vi "四通道零漂采集1A4DEB1.vi"() -> ()   [LabVIEW 2011]
doc: "Use this template to build a producer/consumer design pattern. Use this template when you need to execute a process, such as data analysis, when a data source, such as a triggered acquisition, produces data at an uneven rate and you need to execute the process when the data becomes available."
uses:
  <vilib>/Utility/inputDevices.llb/closeKeyboard.vi
  <vilib>/Utility/inputDevices.llb/keyboardAcquire.vi
  <vilib>/Utility/file.llb/Write To Spreadsheet File (string).vi
  <vilib>/Utility/file.llb/Read From Spreadsheet File (string).vi
  <vilib>/Analysis/NI_AALBase.lvlib
panel:
  in  "每几秒采一个点":i32=1
  in  "计算零偏\n稳定性":bool
  out "零偏值4":dbl[unit]
  out "零偏稳定性4":dbl[unit]
  in  "灵敏度4":dbl[unit]
  out "standard deviation 4":dbl[unit] caption="标准差4" format="%.6f"
  out "mean 4":dbl[unit] caption="平均值4" format="%.6f"
  out "零偏值3":dbl[unit]
  out "零偏稳定性3":dbl[unit]
  in  "灵敏度3":dbl[unit]
  out "standard deviation 3":dbl[unit] caption="标准差3" format="%.6f"
  out "mean 3":dbl[unit] caption="平均值3" format="%.6f"
  out "零偏值2":dbl[unit]
  out "零偏稳定性2":dbl[unit]
  in  "灵敏度2":dbl[unit]
  out "standard deviation 2":dbl[unit] caption="标准差2" format="%.6f"
  out "mean 2":dbl[unit] caption="平均值2" format="%.6f"
  out "零偏值1":dbl[unit]
  out "零偏稳定性1":dbl[unit]
  in  "灵敏度1":dbl[unit]
  out "standard deviation":dbl[unit] caption="标准差1" format="%.6f"
  out "mean":dbl[unit] caption="平均值1" format="%.6f"
  out "0g输出值(V) 3":dbl
  out "0g输出值(V) 2":dbl
  out "0g输出值(V) 1":dbl
  out "a1通道零漂采集":dbl(graph)
  out "a3通道零漂采集":dbl(graph)
  out "a2通道零漂采集":dbl(graph)
  in  "删除文件":bool
  in  "打开文件":bool
  in  "创建文件":bool
  in  "开始采零漂":bool
  in  "打开采集卡":bool
  in  "闹钟定时":bool
  in  "时间标识":timestamp format="%<%H:%M\n%x>T"
  out "采集数据":string[][](array[string])
  out "点数":i16
  out "x":i16
  in  "传感器编号":string
  out "a0通道零漂采集":dbl(graph)
  out "0g输出值(V)":dbl
  in  "stop":bool
  # "四通道零漂采集测试"
  # "D"
  # "O"
  # "N"
  # "S"
  # "B"
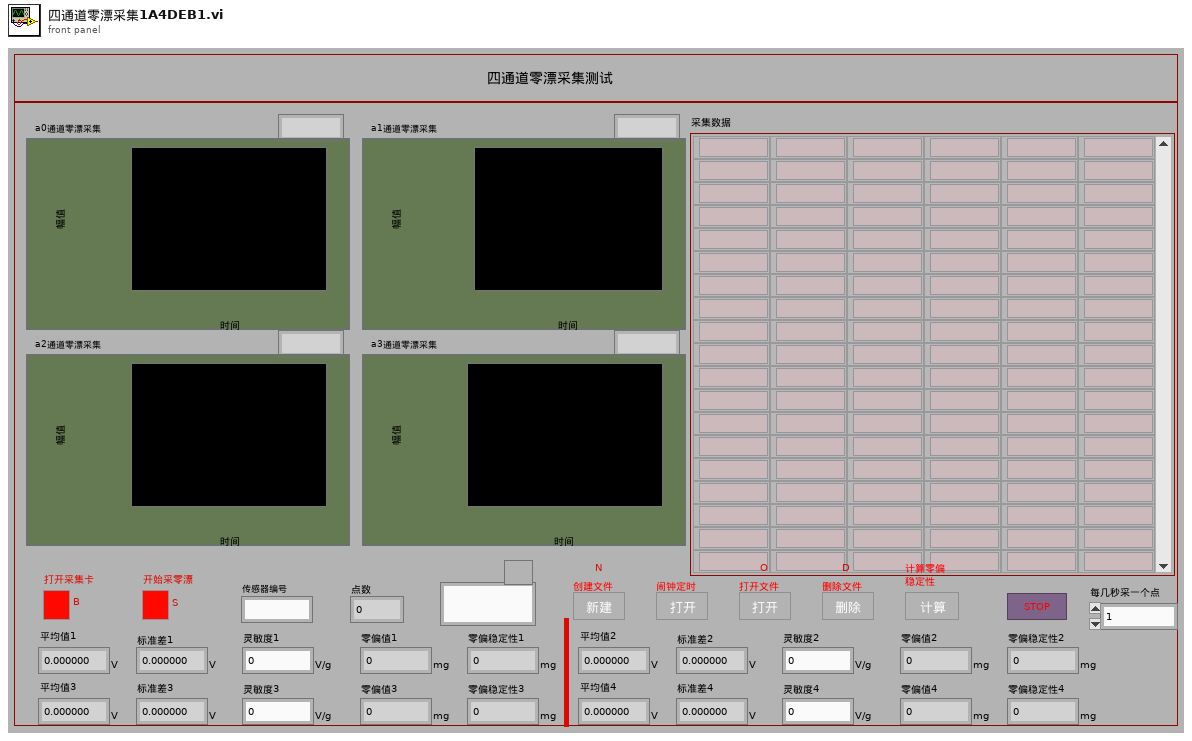
[diagram p1: front panel]
types:
  T1 = enum16{"0", "1", "2", "3", "4", "5", "6", "7", "8", "9", "A", "B", "C", "D", "E", "F", "G", "H", "I", "J", "K", "L", "M", "N", "O", "P", "Q", "R", "S", "T", "U", "V", "W", "X", "Y", "Z", "F1", "F2", "F3", "F4", "F5", "F6", "F7", "F8", "F9", "F10", "F11", "F12", "F13", "F14", "F15", "ADD", "BACK", "BACKSLASH", "CAPITAL", "COMMA", "DECIMAL", "DELETE", "DIVIDE", "DOWN", "END", "EQUALS", "ESCAPE", "GRAVE (`)", "HOME", "INSERT", "LBRACKET", "LCONTROL", "LEFT", "L ALT", "LSHIFT", "LWIN", "MINUS", "MULTIPLY", "NEXT", "NUMLOCK", "NUMPAD_0", "NUMPAD_1", "NUMPAD_2", "NUMPAD_3", "NUMPAD_4", "NUMPAD_5", "NUMPAD_6", "NUMPAD_7", "NUMPAD_8", "NUMPAD_9", "PAUSE", "PERIOD", "PRIOR (PG UP)", "RBRACKET", "RCONTROL", "RETURN", "RIGHT", "R ALT", "RSHIFT", "RWIN", "SCROLL", "SEMICOLON", "SLASH", "SPACE", "SUBTRACT", "TAB", "UP", "ENTER (num pad)", "' (quote)"}
  T2 = enum16{"0", "1", "2", "3", "4", "5", "6", "7", "8", "9", "A", "B", "C", "D", "E", "F", "G", "H", "I", "J", "K", "L", "M", "N", "O", "P", "Q", "R", "S", "T", "U", "V", "W", "X", "Y", "Z", "F1", "F2", "F3", "F4", "F5", "F6", "F7", "F8", "F9", "F10", "F11", "F12", "F13", "F14", "F15", "ADD", "BACK", "BACKSLASH", "CAPITAL", "COMMA", "DECIMAL", "DELETE", "DIVIDE", "DOWN", "END", "EQUALS", "ESCAPE", "GRAVE (`)", "HOME", "INSERT", "LBRACKET", "LCONTROL", "LEFT", "L ALT", "LSHIFT", "LWIN", "MINUS", "MULTIPLY", "NEXT", "NUMLOCK", "NUMPAD_0", "NUMPAD_1", "NUMPAD_2", "NUMPAD_3", "NUMPAD_4", "NUMPAD_5", "NUMPAD_6", "NUMPAD_7", "NUMPAD_8", "NUMPAD_9", "PAUSE", "PERIOD", "PRIOR (PG UP)", "RBRACKET", "RCONTROL", "RETURN", "RIGHT", "R ALT", "RSHIFT", "RWIN", "SCROLL", "SEMICOLON", "SLASH", "SPACE", "SUBTRACT", "TAB", "UP", "ENTER (num pad)", "' (quote)"}[]
  T3 = cluster{"keys pressed[0]":enum16{"0", "1", "2", "3", "4", "5", "6", "7", "8", "9", "A", "B", "C", "D", "E", "F", "G", "H", "I", "J", "K", "L", "M", "N", "O", "P", "Q", "R", "S", "T", "U", "V", "W", "X", "Y", "Z", "F1", "F2", "F3", "F4", "F5", "F6", "F7", "F8", "F9", "F10", "F11", "F12", "F13", "F14", "F15", "ADD", "BACK", "BACKSLASH", "CAPITAL", "COMMA", "DECIMAL", "DELETE", "DIVIDE", "DOWN", "END", "EQUALS", "ESCAPE", "GRAVE (`)", "HOME", "INSERT", "LBRACKET", "LCONTROL", "LEFT", "L ALT", "LSHIFT", "LWIN", "MINUS", "MULTIPLY", "NEXT", "NUMLOCK", "NUMPAD_0", "NUMPAD_1", "NUMPAD_2", "NUMPAD_3", "NUMPAD_4", "NUMPAD_5", "NUMPAD_6", "NUMPAD_7", "NUMPAD_8", "NUMPAD_9", "PAUSE", "PERIOD", "PRIOR (PG UP)", "RBRACKET", "RCONTROL", "RETURN", "RIGHT", "R ALT", "RSHIFT", "RWIN", "SCROLL", "SEMICOLON", "SLASH", "SPACE", "SUBTRACT", "TAB", "UP", "ENTER (num pad)", "' (quote)"}, "keys pressed[1]":enum16{"0", "1", "2", "3", "4", "5", "6", "7", "8", "9", "A", "B", "C", "D", "E", "F", "G", "H", "I", "J", "K", "L", "M", "N", "O", "P", "Q", "R", "S", "T", "U", "V", "W", "X", "Y", "Z", "F1", "F2", "F3", "F4", "F5", "F6", "F7", "F8", "F9", "F10", "F11", "F12", "F13", "F14", "F15", "ADD", "BACK", "BACKSLASH", "CAPITAL", "COMMA", "DECIMAL", "DELETE", "DIVIDE", "DOWN", "END", "EQUALS", "ESCAPE", "GRAVE (`)", "HOME", "INSERT", "LBRACKET", "LCONTROL", "LEFT", "L ALT", "LSHIFT", "LWIN", "MINUS", "MULTIPLY", "NEXT", "NUMLOCK", "NUMPAD_0", "NUMPAD_1", "NUMPAD_2", "NUMPAD_3", "NUMPAD_4", "NUMPAD_5", "NUMPAD_6", "NUMPAD_7", "NUMPAD_8", "NUMPAD_9", "PAUSE", "PERIOD", "PRIOR (PG UP)", "RBRACKET", "RCONTROL", "RETURN", "RIGHT", "R ALT", "RSHIFT", "RWIN", "SCROLL", "SEMICOLON", "SLASH", "SPACE", "SUBTRACT", "TAB", "UP", "ENTER (num pad)", "' (quote)"}, "keys pressed[2]":enum16{"0", "1", "2", "3", "4", "5", "6", "7", "8", "9", "A", "B", "C", "D", "E", "F", "G", "H", "I", "J", "K", "L", "M", "N", "O", "P", "Q", "R", "S", "T", "U", "V", "W", "X", "Y", "Z", "F1", "F2", "F3", "F4", "F5", "F6", "F7", "F8", "F9", "F10", "F11", "F12", "F13", "F14", "F15", "ADD", "BACK", "BACKSLASH", "CAPITAL", "COMMA", "DECIMAL", "DELETE", "DIVIDE", "DOWN", "END", "EQUALS", "ESCAPE", "GRAVE (`)", "HOME", "INSERT", "LBRACKET", "LCONTROL", "LEFT", "L ALT", "LSHIFT", "LWIN", "MINUS", "MULTIPLY", "NEXT", "NUMLOCK", "NUMPAD_0", "NUMPAD_1", "NUMPAD_2", "NUMPAD_3", "NUMPAD_4", "NUMPAD_5", "NUMPAD_6", "NUMPAD_7", "NUMPAD_8", "NUMPAD_9", "PAUSE", "PERIOD", "PRIOR (PG UP)", "RBRACKET", "RCONTROL", "RETURN", "RIGHT", "R ALT", "RSHIFT", "RWIN", "SCROLL", "SEMICOLON", "SLASH", "SPACE", "SUBTRACT", "TAB", "UP", "ENTER (num pad)", "' (quote)"}, "keys pressed[3]":enum16{"0", "1", "2", "3", "4", "5", "6", "7", "8", "9", "A", "B", "C", "D", "E", "F", "G", "H", "I", "J", "K", "L", "M", "N", "O", "P", "Q", "R", "S", "T", "U", "V", "W", "X", "Y", "Z", "F1", "F2", "F3", "F4", "F5", "F6", "F7", "F8", "F9", "F10", "F11", "F12", "F13", "F14", "F15", "ADD", "BACK", "BACKSLASH", "CAPITAL", "COMMA", "DECIMAL", "DELETE", "DIVIDE", "DOWN", "END", "EQUALS", "ESCAPE", "GRAVE (`)", "HOME", "INSERT", "LBRACKET", "LCONTROL", "LEFT", "L ALT", "LSHIFT", "LWIN", "MINUS", "MULTIPLY", "NEXT", "NUMLOCK", "NUMPAD_0", "NUMPAD_1", "NUMPAD_2", "NUMPAD_3", "NUMPAD_4", "NUMPAD_5", "NUMPAD_6", "NUMPAD_7", "NUMPAD_8", "NUMPAD_9", "PAUSE", "PERIOD", "PRIOR (PG UP)", "RBRACKET", "RCONTROL", "RETURN", "RIGHT", "R ALT", "RSHIFT", "RWIN", "SCROLL", "SEMICOLON", "SLASH", "SPACE", "SUBTRACT", "TAB", "UP", "ENTER (num pad)", "' (quote)"}, "keys pressed[4]":enum16{"0", "1", "2", "3", "4", "5", "6", "7", "8", "9", "A", "B", "C", "D", "E", "F", "G", "H", "I", "J", "K", "L", "M", "N", "O", "P", "Q", "R", "S", "T", "U", "V", "W", "X", "Y", "Z", "F1", "F2", "F3", "F4", "F5", "F6", "F7", "F8", "F9", "F10", "F11", "F12", "F13", "F14", "F15", "ADD", "BACK", "BACKSLASH", "CAPITAL", "COMMA", "DECIMAL", "DELETE", "DIVIDE", "DOWN", "END", "EQUALS", "ESCAPE", "GRAVE (`)", "HOME", "INSERT", "LBRACKET", "LCONTROL", "LEFT", "L ALT", "LSHIFT", "LWIN", "MINUS", "MULTIPLY", "NEXT", "NUMLOCK", "NUMPAD_0", "NUMPAD_1", "NUMPAD_2", "NUMPAD_3", "NUMPAD_4", "NUMPAD_5", "NUMPAD_6", "NUMPAD_7", "NUMPAD_8", "NUMPAD_9", "PAUSE", "PERIOD", "PRIOR (PG UP)", "RBRACKET", "RCONTROL", "RETURN", "RIGHT", "R ALT", "RSHIFT", "RWIN", "SCROLL", "SEMICOLON", "SLASH", "SPACE", "SUBTRACT", "TAB", "UP", "ENTER (num pad)", "' (quote)"}, "keys pressed[5]":enum16{"0", "1", "2", "3", "4", "5", "6", "7", "8", "9", "A", "B", "C", "D", "E", "F", "G", "H", "I", "J", "K", "L", "M", "N", "O", "P", "Q", "R", "S", "T", "U", "V", "W", "X", "Y", "Z", "F1", "F2", "F3", "F4", "F5", "F6", "F7", "F8", "F9", "F10", "F11", "F12", "F13", "F14", "F15", "ADD", "BACK", "BACKSLASH", "CAPITAL", "COMMA", "DECIMAL", "DELETE", "DIVIDE", "DOWN", "END", "EQUALS", "ESCAPE", "GRAVE (`)", "HOME", "INSERT", "LBRACKET", "LCONTROL", "LEFT", "L ALT", "LSHIFT", "LWIN", "MINUS", "MULTIPLY", "NEXT", "NUMLOCK", "NUMPAD_0", "NUMPAD_1", "NUMPAD_2", "NUMPAD_3", "NUMPAD_4", "NUMPAD_5", "NUMPAD_6", "NUMPAD_7", "NUMPAD_8", "NUMPAD_9", "PAUSE", "PERIOD", "PRIOR (PG UP)", "RBRACKET", "RCONTROL", "RETURN", "RIGHT", "R ALT", "RSHIFT", "RWIN", "SCROLL", "SEMICOLON", "SLASH", "SPACE", "SUBTRACT", "TAB", "UP", "ENTER (num pad)", "' (quote)"}, "keys pressed[6]":enum16{"0", "1", "2", "3", "4", "5", "6", "7", "8", "9", "A", "B", "C", "D", "E", "F", "G", "H", "I", "J", "K", "L", "M", "N", "O", "P", "Q", "R", "S", "T", "U", "V", "W", "X", "Y", "Z", "F1", "F2", "F3", "F4", "F5", "F6", "F7", "F8", "F9", "F10", "F11", "F12", "F13", "F14", "F15", "ADD", "BACK", "BACKSLASH", "CAPITAL", "COMMA", "DECIMAL", "DELETE", "DIVIDE", "DOWN", "END", "EQUALS", "ESCAPE", "GRAVE (`)", "HOME", "INSERT", "LBRACKET", "LCONTROL", "LEFT", "L ALT", "LSHIFT", "LWIN", "MINUS", "MULTIPLY", "NEXT", "NUMLOCK", "NUMPAD_0", "NUMPAD_1", "NUMPAD_2", "NUMPAD_3", "NUMPAD_4", "NUMPAD_5", "NUMPAD_6", "NUMPAD_7", "NUMPAD_8", "NUMPAD_9", "PAUSE", "PERIOD", "PRIOR (PG UP)", "RBRACKET", "RCONTROL", "RETURN", "RIGHT", "R ALT", "RSHIFT", "RWIN", "SCROLL", "SEMICOLON", "SLASH", "SPACE", "SUBTRACT", "TAB", "UP", "ENTER (num pad)", "' (quote)"}, "keys pressed[7]":enum16{"0", "1", "2", "3", "4", "5", "6", "7", "8", "9", "A", "B", "C", "D", "E", "F", "G", "H", "I", "J", "K", "L", "M", "N", "O", "P", "Q", "R", "S", "T", "U", "V", "W", "X", "Y", "Z", "F1", "F2", "F3", "F4", "F5", "F6", "F7", "F8", "F9", "F10", "F11", "F12", "F13", "F14", "F15", "ADD", "BACK", "BACKSLASH", "CAPITAL", "COMMA", "DECIMAL", "DELETE", "DIVIDE", "DOWN", "END", "EQUALS", "ESCAPE", "GRAVE (`)", "HOME", "INSERT", "LBRACKET", "LCONTROL", "LEFT", "L ALT", "LSHIFT", "LWIN", "MINUS", "MULTIPLY", "NEXT", "NUMLOCK", "NUMPAD_0", "NUMPAD_1", "NUMPAD_2", "NUMPAD_3", "NUMPAD_4", "NUMPAD_5", "NUMPAD_6", "NUMPAD_7", "NUMPAD_8", "NUMPAD_9", "PAUSE", "PERIOD", "PRIOR (PG UP)", "RBRACKET", "RCONTROL", "RETURN", "RIGHT", "R ALT", "RSHIFT", "RWIN", "SCROLL", "SEMICOLON", "SLASH", "SPACE", "SUBTRACT", "TAB", "UP", "ENTER (num pad)", "' (quote)"}, "keys pressed[8]":enum16{"0", "1", "2", "3", "4", "5", "6", "7", "8", "9", "A", "B", "C", "D", "E", "F", "G", "H", "I", "J", "K", "L", "M", "N", "O", "P", "Q", "R", "S", "T", "U", "V", "W", "X", "Y", "Z", "F1", "F2", "F3", "F4", "F5", "F6", "F7", "F8", "F9", "F10", "F11", "F12", "F13", "F14", "F15", "ADD", "BACK", "BACKSLASH", "CAPITAL", "COMMA", "DECIMAL", "DELETE", "DIVIDE", "DOWN", "END", "EQUALS", "ESCAPE", "GRAVE (`)", "HOME", "INSERT", "LBRACKET", "LCONTROL", "LEFT", "L ALT", "LSHIFT", "LWIN", "MINUS", "MULTIPLY", "NEXT", "NUMLOCK", "NUMPAD_0", "NUMPAD_1", "NUMPAD_2", "NUMPAD_3", "NUMPAD_4", "NUMPAD_5", "NUMPAD_6", "NUMPAD_7", "NUMPAD_8", "NUMPAD_9", "PAUSE", "PERIOD", "PRIOR (PG UP)", "RBRACKET", "RCONTROL", "RETURN", "RIGHT", "R ALT", "RSHIFT", "RWIN", "SCROLL", "SEMICOLON", "SLASH", "SPACE", "SUBTRACT", "TAB", "UP", "ENTER (num pad)", "' (quote)"}}
  T4 = typedef "LVDateTimeRec.ctl" = cluster{"秒数的小数部分":dbl, "秒":i32, "分":i32, "小时":i32, "每月天数":i32, "月":i32, "年":i32, "每周天数":i32, "每年天数":i32, "离散正弦变换":i32}
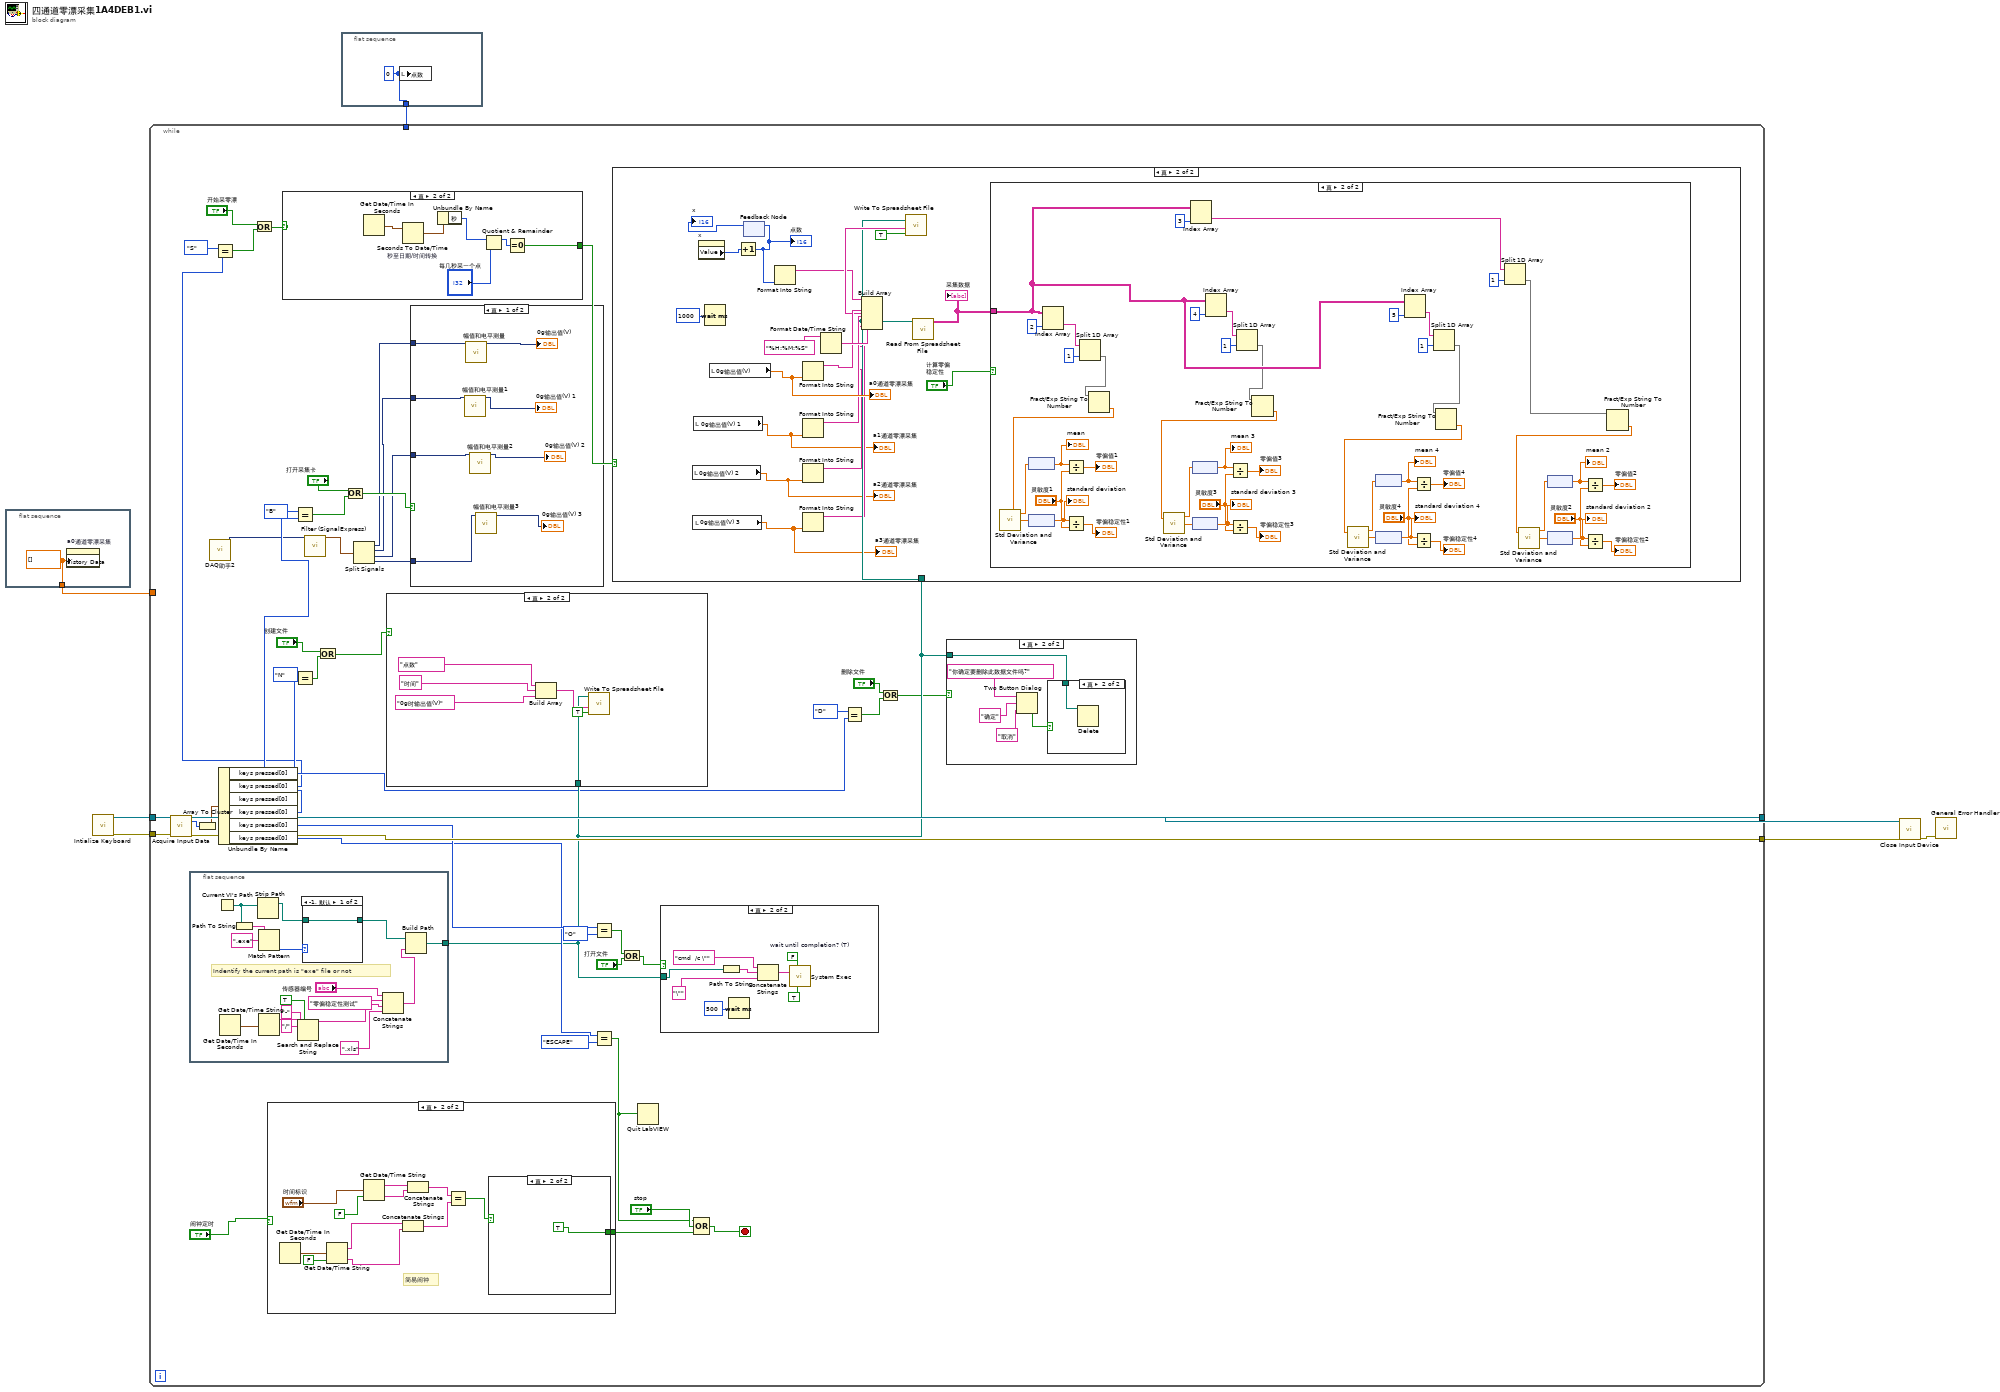
[diagram p0: block diagram]
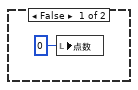
[diagram p6: hidden frame]
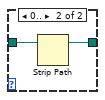
[diagram p8: hidden frame]
diagram:
  n1 = flat-sequence {
    tunnel: [w8] -> w7
    frame #0 {
      w8 = dbl[] [] ("历史数据")
      n2 = property on="a0通道零漂采集" class="WFChart (严格)"("History Data"=w8) -> ()  [unwired: 2 in, 2 out]
    }
  }
  n3 = call <vilib>:"Intialize Keyboard.vi"() -> ("error out"=w3:errorcluster, "device ID"=w4:refnum<k1>)  [unwired: 10 in]
  n4 = while {
    tunnel: w7 -> [_]
    tunnel: [w53] -> w5
    tunnel: w4 -> [w52]
    tunnel: w3 -> [w51]
    tunnel: [w50] -> w2
    tunnel: w1 -> [_]
    stop <- w24 stop-if-true
    n5 = call-poly <vilib>:"Acquire Input Data.vi"("device ID"=w52, "error in (no error)"=w51) -> ("device ID"=w53:refnum<k1>, "keys pressed"=w49:T2, "error out"=w50:errorcluster)  [unwired: 15 in]
    n6 = flat-sequence {
      tunnel: [w89] -> w21
      frame #0 {
        # "Indentify the current path is \"exe\" file or not"
        n7 = Current VI's Path() -> (path=w104:path)
        n8 = Get Date/Time In Seconds() -> (seconds since 1Jan1904=w96:timestamp)
        n9 = Path To String(path=w104) -> (string=w105:string)
        n10 = Strip Path(path=w104) -> (stripped path=w101:path)  [unwired: 1 out]
        n11 = Match Pattern(string=w105, regular expression=".exe") -> (offset past match=w102:i32)  [unwired: 1 in, 3 out]
        n12 = Get Date/Time String(seconds (now)=w96) -> (date string=w95:string)  [unwired: 2 in, 1 out]
        n13 = Search and Replace String(replace all?=TRUE ("替换全部？(F)"), input string=w95, search string="/" ("搜索字符串"), replace string="-" ("替换字符串(\"\")")) -> (result string=w91:string)  [unwired: 4 in, 3 out]
        n14 = case shown="-1, 默认" w102 {
          tunnel: [w106 w108] -> w100
          tunnel: w101 -> [w106 w107]
          frame -1, Default {
          }
          frame 0.. {
            n15 = Strip Path(path=w107) -> (stripped path=w108:path)  [unwired: 1 out]
          }
        }
        n16 = Concatenate Strings("传感器编号", "零偏稳定性测试", w91, ".xls") -> (w97:string)
        n17 = Build Path(base path=w100, name or relative path=w97) -> (appended path=w89:path)
      }
    }
    n18 = Array To Cluster(array=w49) -> (cluster=w48:T3)
    n19 = call "DAQ助手2"() -> ("data"=w15:dynamicdata)  [unwired: 16 in, 3 out]
    n20 = Unbundle By Name(w48) -> ("keys pressed[0]"=w17:T1, "keys pressed[0]"=w9:T1, "keys pressed[0]"=w39:T1, "keys pressed[0]"=w47:T1, "keys pressed[0]"=w30:T1, "keys pressed[0]"=w22:T1)
    n21 = Equal?(x=T1."S", y=w9) -> (x = y?=w35:bool)
    n22 = Or(x="开始采零漂", y=w35) -> (x .or. y?=w37:bool)
    n23 = case shown="真" "闹钟定时" {
      tunnel: [_ w61] -> w28
      frame False {
      }
      frame True {
        # "简易闹钟"
        n24 = Get Date/Time In Seconds() -> (seconds since 1Jan1904=w64:timestamp)
        n25 = Get Date/Time String(seconds (now)=w64, want seconds? (F)=FALSE) -> (date string=w65:string, time string=w66:string)  [unwired: 1 in]
        n26 = Get Date/Time String(seconds (now)="时间标识", want seconds? (F)=FALSE) -> (date string=w68:string, time string=w69:string)  [unwired: 1 in]
        n27 = Concatenate Strings(w65, w66) -> (w71:string)
        n28 = Concatenate Strings(w68, w69) -> (w70:string)
        n29 = Equal?(x=w70, y=w71) -> (x = y?=w72:bool)
        n30 = case shown="真" w72 {
          tunnel: [_ TRUE] -> w61
          frame False {
          }
          frame True {
          }
        }
      }
    }
    n31 = case shown="真" w37 {
      tunnel: [_ w76] -> w54
      frame False {
        n32 = local write "点数"(i16 0 ("点数")) -> ()
      }
      frame True {
        n33 = Get Date/Time In Seconds() -> (seconds since 1Jan1904=w80:timestamp)
        n34 = Seconds To Date/Time "秒至日期/时间转换"(time stamp (now)=w80) -> (date time rec=w79:T4)  [unwired: 1 in]
        n35 = Unbundle By Name ("按名称解除捆绑")(w79) -> ("秒"=w78:i32)
        n36 = Quotient & Remainder(x=w78, y="每几秒采一个点") -> (x-y*floor(x/y)=w77:i32)  [unwired: 1 out]
        n37 = Equal To 0?(x=w77) -> (x = 0?=w76:bool)
      }
    }
    n38 = Equal?(x=T1."B", y=w39) -> (x = y?=w41:bool)
    n39 = Equal?(x=T1."N", y=w47) -> (x = y?=w44:bool)
    n40 = call "Filter (SignalExpress)"("input signals"=w15) -> ("filtered data"=w14:waveform(dbl)[])  [unwired: 17 in, 1 out]
    n41 = Or(x="创建文件", y=w44) -> (x .or. y?=w43:bool)
    n42 = Or(x="打开采集卡", y=w41) -> (x .or. y?=w40:bool)
    n43 = Split Signals(w14) -> (w13:dynamicdata, w12:dynamicdata, w11:dynamicdata, w10:dynamicdata)  [unwired: 4 in]
    n44 = case shown="真" w43 {
      tunnel: w21 -> [_ w179]
      frame False {
      }
      frame True {
        n45 = Build Array("点数", "时间", "0g时输出值(V)") -> (w180:string[])
        n46 = call-poly <vilib>:"Write To Spreadsheet File.vi"("append to file? (new file:F)"=TRUE, "1D data"=w180, "file path (dialog if empty)"=w179) -> ()  [unwired: 5 in, 1 out]
      }
    }
    n47 = case shown="真" w40 {
      tunnel: w13 -> [w187 _]
      tunnel: w12 -> [w186 _]
      tunnel: w11 -> [w185 _]
      tunnel: w10 -> [w184 _]
      frame True {
        n48 = call "幅值和电平测量1"("Signals"=w186) -> ("Mean (DC)"=→"0g输出值(V) 1":dynamicdata)  [unwired: 13 in, 1 out]
        n49 = call "幅值和电平测量"("Signals"=w187) -> ("Mean (DC)"=→"0g输出值(V)":dynamicdata)  [unwired: 13 in, 1 out]
        n50 = call "幅值和电平测量2"("Signals"=w185) -> ("Mean (DC)"=→"0g输出值(V) 2":dynamicdata)  [unwired: 13 in, 1 out]
        n51 = call "幅值和电平测量3"("Signals"=w184) -> ("Mean (DC)"=→"0g输出值(V) 3":dynamicdata)  [unwired: 13 in, 1 out]
      }
      frame False {
      }
    }
    n52 = Equal?(x=w30, y=T1."O") -> (x = y?=w31:bool)
    n53 = Equal?(x=w22, y=T1."ESCAPE") -> (x = y?=w25:bool)
    n54 = case shown="真" w54 {
      tunnel: w21 -> [_ w122]
      frame False {
      }
      frame True {
        n55 = local read "0g输出值(V) 2"() -> (w112:dbl)
        "a2通道零漂采集" <- w112
        n56 = local read "0g输出值(V) 3"() -> (w111:dbl)
        "a3通道零漂采集" <- w111
        n57 = local read "0g输出值(V) 1"() -> (w113:dbl)
        "a1通道零漂采集" <- w113
        n58 = property on="x" class="DigNum (严格)"() -> ("Value"=w118:i16)  [unwired: 2 in, 2 out]
        n59 = Wait (ms)(milliseconds to wait=u32 1000 ("等待时间（毫秒）")) -> ()  [unwired: 1 out]
        n60 = local read "0g输出值(V)"() -> (w123:dbl)
        "a0通道零漂采集" <- w123
        n61 = Increment(x=w118) -> (x+1=w119:i16)
        "点数" <- w119
        n62 = feedback-in #1(w119) -> ()
        n63 = feedback #1() -> (→"x":i16)  [unwired: 1 in]
        n64 = Format Into String(w119) -> (resulting string=w120:string)  [unwired: 3 in, 1 out]
        n65 = Format Into String(w123) -> (resulting string=w125:string)  [unwired: 3 in, 1 out]
        n66 = Format Into String(w113) -> (resulting string=w116:string)  [unwired: 3 in, 1 out]
        n67 = Format Into String(w112) -> (resulting string=w115:string)  [unwired: 3 in, 1 out]
        n68 = Format Into String(w111) -> (resulting string=w114:string)  [unwired: 3 in, 1 out]
        n69 = Format Date/Time String(time format string (%c)="%H:%M:%S") -> (date/time string=w126:string)  [unwired: 2 in]
        n70 = Build Array(w120, w126, w125, w116, w115, w114) -> (w124:string[])
        n71 = call-poly <vilib>:"Write To Spreadsheet File.vi"("append to file? (new file:F)"=TRUE, "1D data"=w124, "file path (dialog if empty)"=w122) -> ()  [unwired: 5 in, 1 out]
        n72 = call-poly <vilib>:"Read From Spreadsheet File.vi"("file path (dialog if empty)"=w122) -> ("all rows"=w110:string[][])  [unwired: 6 in, 4 out]
        "采集数据" <- w110
        n73 = case shown="真" "计算零偏\n稳定性" {
          tunnel: w110 -> [_ w142]
          frame False {
          }
          frame True {
            n74 = Index Array(array=w142, index (col)=2 ("禁用的索引 (列)")) -> (element=w136:string[])  [unwired: 1 in]
            n75 = Split 1D Array(array=w136, index=1 ("索引")) -> (second subarray=w135:string[])  [unwired: 1 out]
            n76 = Fract/Exp String To Number(string=w135) -> (number=w169:dbl[])  [unwired: 3 in, 1 out]
            n77 = call <vilib>:"Std Deviation and Variance.vi"("X"=w169) -> ("mean"=w177:dbl, "standard deviation"=w176:dbl)  [unwired: 1 in, 1 out]
            n78 = node(w177) -> (w173:dbl[unit])
            "mean" <- w173
            n79 = node(w176) -> (w175:dbl[unit])
            "standard deviation" <- w175
            n80 = Divide(x=w173, y="灵敏度1") -> (x/y=→"零偏值1":dbl[unit])
            n81 = Divide(x=w175, y="灵敏度1") -> (x/y=→"零偏稳定性1":dbl[unit])
            n82 = Index Array(array=w142, index (col)=3 ("禁用的索引 (列)")) -> (element=w130:string[])  [unwired: 1 in]
            n83 = Index Array(array=w142, index (col)=4 ("禁用的索引 (列)")) -> (element=w134:string[])  [unwired: 1 in]
            n84 = Split 1D Array(array=w134, index=1 ("索引")) -> (second subarray=w133:string[])  [unwired: 1 out]
            n85 = Fract/Exp String To Number(string=w133) -> (number=w151:dbl[])  [unwired: 3 in, 1 out]
            n86 = call <vilib>:"Std Deviation and Variance.vi"("X"=w151) -> ("mean"=w159:dbl, "standard deviation"=w158:dbl)  [unwired: 1 in, 1 out]
            n87 = node(w159) -> (w155:dbl[unit])
            "mean 3" <- w155
            n88 = node(w158) -> (w157:dbl[unit])
            "standard deviation 3" <- w157
            n89 = Divide(x=w155, y="灵敏度3") -> (x/y=→"零偏值3":dbl[unit])
            n90 = Divide(x=w157, y="灵敏度3") -> (x/y=→"零偏稳定性3":dbl[unit])
            n91 = Index Array(array=w142, index (col)=5 ("禁用的索引 (列)")) -> (element=w132:string[])  [unwired: 1 in]
            n92 = Split 1D Array(array=w132, index=1 ("索引")) -> (second subarray=w131:string[])  [unwired: 1 out]
            n93 = Fract/Exp String To Number(string=w131) -> (number=w141:dbl[])  [unwired: 3 in, 1 out]
            n94 = call <vilib>:"Std Deviation and Variance.vi"("X"=w141) -> ("mean"=w150:dbl, "standard deviation"=w149:dbl)  [unwired: 1 in, 1 out]
            n95 = node(w150) -> (w146:dbl[unit])
            "mean 4" <- w146
            n96 = node(w149) -> (w148:dbl[unit])
            "standard deviation 4" <- w148
            n97 = Divide(x=w146, y="灵敏度4") -> (x/y=→"零偏值4":dbl[unit])
            n98 = Divide(x=w148, y="灵敏度4") -> (x/y=→"零偏稳定性4":dbl[unit])
            n99 = Split 1D Array(array=w130, index=1 ("索引")) -> (second subarray=w129:string[])  [unwired: 1 out]
            n100 = Fract/Exp String To Number(string=w129) -> (number=w160:dbl[])  [unwired: 3 in, 1 out]
            n101 = call <vilib>:"Std Deviation and Variance.vi"("X"=w160) -> ("mean"=w168:dbl, "standard deviation"=w167:dbl)  [unwired: 1 in, 1 out]
            n102 = node(w168) -> (w164:dbl[unit])
            "mean 2" <- w164
            n103 = node(w167) -> (w166:dbl[unit])
            "standard deviation 2" <- w166
            n104 = Divide(x=w164, y="灵敏度2") -> (x/y=→"零偏值2":dbl[unit])
            n105 = Divide(x=w166, y="灵敏度2") -> (x/y=→"零偏稳定性2":dbl[unit])
          }
        }
      }
    }
    n106 = Or(x=w31, y="打开文件") -> (x .or. y?=w33:bool)
    n107 = Quit LabVIEW(quit? (T)=w25) -> ()
    n108 = case shown="真" w33 {
      tunnel: w21 -> [_ w81]
      frame False {
      }
      frame True {
        w88 = FALSE  # wait until completion? (T)
        n109 = Path To String(path=w81) -> (string=w85:string)
        n110 = Wait (ms)(milliseconds to wait=u32 500 ("等待时间（毫秒）")) -> ()  [unwired: 1 out]
        n111 = Concatenate Strings("cmd  /c \"", w85, "\"") -> (w83:string)
        n112 = call <vilib>:"System Exec.vi"("run minimized? (F)"=TRUE, "wait until completion? (T)"=w88, "command line"=w83) -> ()  [unwired: 3 in, 6 out]
      }
    }
    n113 = Compound Arithmetic op=OR(w25, "stop", w28) -> (w24:bool)
    n114 = Equal?(x=T1."D", y=w17) -> (x = y?=w18:bool)
    n115 = Or(x="删除文件", y=w18) -> (x .or. y?=w20:bool)
    n116 = case shown="真" w20 {
      tunnel: w21 -> [_ w55]
      frame False {
      }
      frame True {
        n117 = Two Button Dialog(message="你确定要删除此数据文件吗?", 1:"取消" ("F button name (\"Cancel\")"), 2:"确定" ("T button name (\"OK\")")) -> (T button?=w59:bool)
        n118 = case shown="真" w59 {
          tunnel: w55 -> [_ w60]
          frame False {
          }
          frame True {
            n119 = Delete(path (use dialog)=w60) -> ()  [unwired: 4 in, 3 out]
          }
        }
      }
    }
  }
  n120 = flat-sequence {
    tunnel: [w192] -> w1
    frame #0 {
      w192 = i16 0 ("点数")
      n121 = local write "点数"(w192) -> ()
    }
  }
  n122 = call-poly <vilib>:"Close Input Device.vi"("error in (no error)"=w2, "device ID"=w5) -> ("error out"=w6:errorcluster)  [unwired: 8 in]
  n123 = call <vilib>:"General Error Handler.vi"("error in (no error)"=w6) -> ()  [unwired: 10 in, 5 out]
